vi "CMD_FITCIRCLE.vi"(6 "Gantry in":refnum<class "Gantry.lvclass">, 8 "error in (no error)":errorcluster, 10 "Arguments":string[](array[string]), 11 "gScript Interpreter in":refnum<class "gScript Interpreter.lvclass">) -> (0 "error out":errorcluster, 3 "gScript Interpreter out":refnum<class "gScript Interpreter.lvclass">, 4 "Gantry out":refnum<class "Gantry.lvclass">)   [LabVIEW 2024, in "gScript Interpreter.lvclass"]
uses:
  gScript Interpreter.lvclass
  Shared Components/Gantry Class/Gantry.lvclass
  Shared Components/Vec3d Class/Vec3d.lvclass
panel:
  in  "Continue":bool
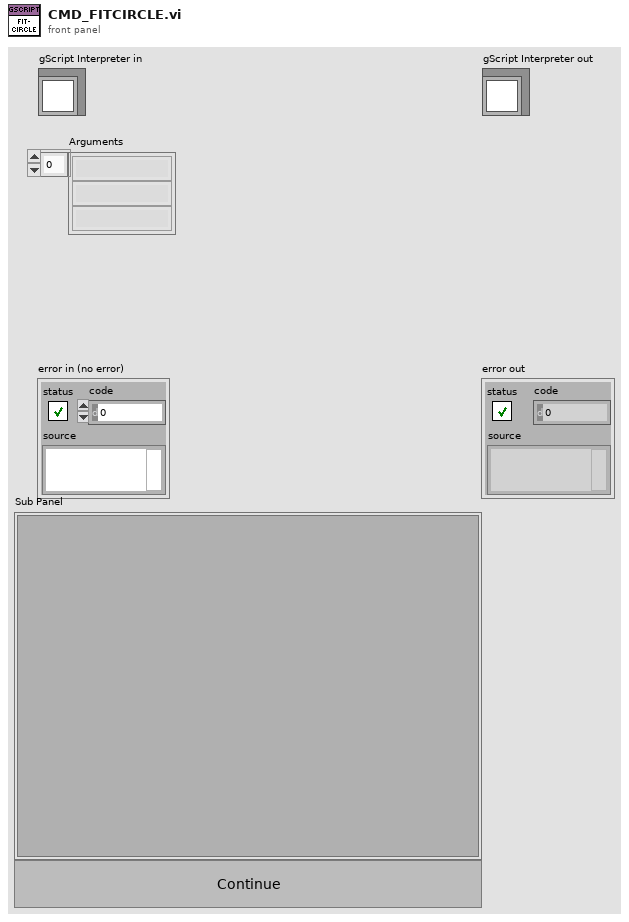
[diagram p1: front panel]
types:
  T1 = typedef "Memory Cell.ctl" = cluster{"type":T2, "x":dbl, "y":dbl, "z":dbl, "w":dbl}
  T2 = typedef "Memory Cell Type Enum.ctl" = enum16{"integer", "float", "vector", "rotation"}
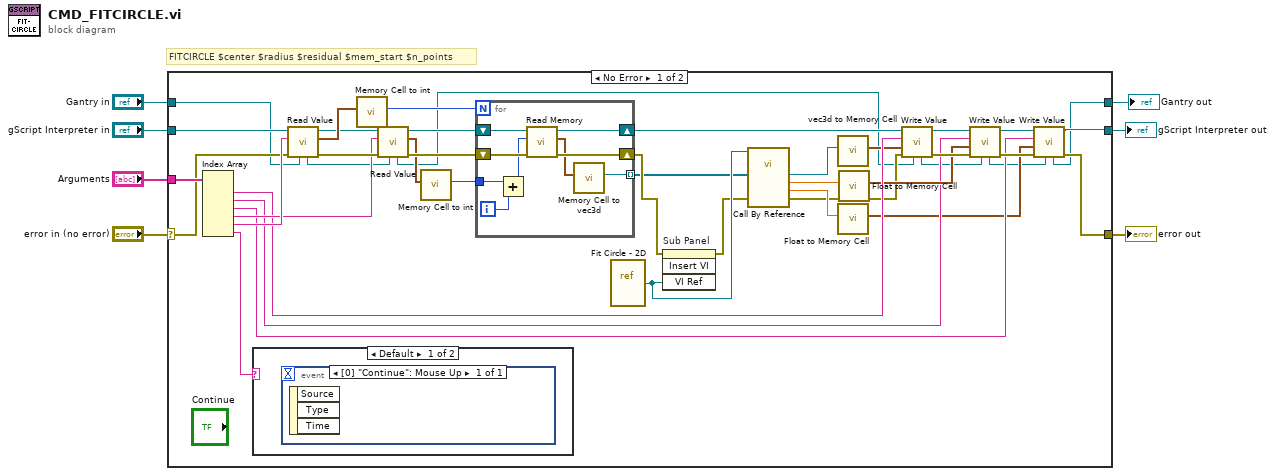
[diagram p0: block diagram]
diagram:
  # "FITCIRCLE $center $radius $residual $mem_start $n_points"
  n1 = case shown="No Error" "error in (no error)" {
    selector: "error in (no error)" -> [w45 w60]
    tunnel: [w23 w60] -> w6
    tunnel: [w24 w59] -> w4
    tunnel: "gScript Interpreter in" -> [w47 w59]
    tunnel: "Arguments" -> [w48 _]
    tunnel: "Gantry in" -> [w13 w58]
    tunnel: [w8 w58] -> w1
    frame No Error {
      n2 = Index Array(array=w48) -> (element #1=w30:string, element #2=w27:string, element #3=w26:string, element #4=w40:string, element #5=w46:string, element #6=w14:string)  [unwired: 6 in]
      n3 = case shown="Default" w14 {
        frame Default {
          n4 = event shown="[0] \"Continue\": Mouse Up" {
            selector: _ -> [_]
            dyn-events: _ -> [_]
            timeout: _ -> [_]
            event "Continue": Mouse Up {
              n5 = event-data() -> ()  [unwired: 1 in, 3 out]
            }
          }
        }
        frame "autoclose" {
        }
      }
      n6 = call-dynamic "Read Value.vi"("Gantry in"=w13, "error in (no error)"=w45, "String in"=w46, "gScript Interpreter in"=w47) -> ("error out"=w41:errorcluster, "Memory Cell"=w44:T1, "gScript Interpreter out"=w42:refnum<class "gScript Interpreter.lvclass">, "Gantry out"=w12:refnum<class "Gantry.lvclass">)  [unwired: 4 in]
      n7 = call "Memory Cell to int.vi"("Memory Cell"=w44) -> ("Int out"=w43:i32)  [unwired: 10 in]
      n8 = call-dynamic "Read Value.vi"("Gantry in"=w12, "error in (no error)"=w41, "String in"=w40, "gScript Interpreter in"=w42) -> ("error out"=w38:errorcluster, "Memory Cell"=w37:T1, "gScript Interpreter out"=w39:refnum<class "gScript Interpreter.lvclass">, "Gantry out"=w11:refnum<class "Gantry.lvclass">)  [unwired: 4 in]
      n9 = call "Memory Cell to int.vi"("Memory Cell"=w37) -> ("Int out"=w36:i32)  [unwired: 10 in]
      n10 = for {
        N: w43 -> [_]
        shift-right: [w56] -> w35
        shift-left: w39 -> [w57]
        shift-right: [w54] -> w22
        shift-left: w38 -> [w55]
        tunnel: [w52] -> w19 mode=indexing
        tunnel: w36 -> [w50]
        i -> [w51]
        n11 = Add(x=w50, y=w51) -> (x+y=w49:i32)
        n12 = call-dynamic "Read Memory.vi"("error in (no error)"=w55, "Memory Address"=w49, "gScript Interpreter in"=w57) -> ("error out"=w54:errorcluster, "Memory Cell"=w53:T1, "gScript Interpreter out"=w56:refnum<class "gScript Interpreter.lvclass">)  [unwired: 6 in]
        n13 = call "Memory Cell to vec3d.vi"("Memory Cell"=w53) -> ("Vec3d out"=w52:refnum<class "Vec3d.lvclass">)  [unwired: 10 in]
      }
      n14 = vi-ref "Fit Circle - 2D.vi"() -> (w21:refnum<vi>)
      n15 = invoke on="Sub Panel" class="SubPnl" method="Insert VI"(error in=w22, "VI Ref"=w21) -> (error out=w20:errorcluster)  [unwired: 2 in, 3 out]
      n16 = call-by-ref "?"(reference=w21, "error in (no error)"=w20, "Points"=w19) -> ("error out"=w15:errorcluster, "Residual"=w16:dbl, "Radius"=w17:dbl, "Center"=w18:refnum<class "Vec3d.lvclass">)  [unwired: 7 in, 2 out]
      n17 = call "vec3d to Memory Cell.vi"("Vec3d in"=w18) -> ("Memory Cell"=w29:T1)  [unwired: 10 in]
      n18 = call "Float to Memory Cell.vi"("Float in"=w16) -> ("Memory Cell"=w25:T1)  [unwired: 10 in]
      n19 = call "Float to Memory Cell.vi"("Float in"=w17) -> ("Memory Cell"=w28:T1)  [unwired: 10 in]
      n20 = call-dynamic "Write Value.vi"("Gantry in"=w11, "error in (no error)"=w15, "Value"=w29, "Address"=w30, "gScript Interpreter in"=w35) -> ("error out"=w32:errorcluster, "gScript Interpreter out"=w34:refnum<class "gScript Interpreter.lvclass">, "Gantry out"=w10:refnum<class "Gantry.lvclass">)  [unwired: 4 in]
      n21 = call-dynamic "Write Value.vi"("Gantry in"=w10, "error in (no error)"=w32, "Value"=w28, "Address"=w27, "gScript Interpreter in"=w34) -> ("error out"=w31:errorcluster, "gScript Interpreter out"=w33:refnum<class "gScript Interpreter.lvclass">, "Gantry out"=w9:refnum<class "Gantry.lvclass">)  [unwired: 4 in]
      n22 = call-dynamic "Write Value.vi"("Gantry in"=w9, "error in (no error)"=w31, "Value"=w25, "Address"=w26, "gScript Interpreter in"=w33) -> ("error out"=w23:errorcluster, "gScript Interpreter out"=w24:refnum<class "gScript Interpreter.lvclass">, "Gantry out"=w8:refnum<class "Gantry.lvclass">)  [unwired: 4 in]
    }
    frame Error {
    }
  }
  "error out" <- w6
  "gScript Interpreter out" <- w4
  "Gantry out" <- w1
